vi "Read.vi"(8 "error in (no error)":errorcluster, 9 "Character Count":u32, 11 "VISA resource name in":refnum<visa-resource-name>) -> (0 "error out":errorcluster, 2 "Characters Read":string, 3 "VISA resource name out":refnum<visa-resource-name>)   [LabVIEW 2021, in "UART.lvlib"]
uses:
  <vilib>/myRIO/Instrument Drivers/Onboard IO/UART/UART.lvlib
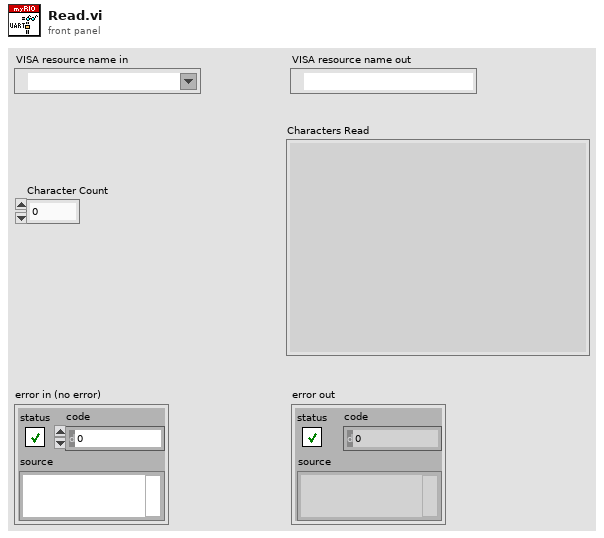
[diagram p1: front panel]
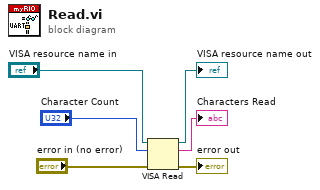
[diagram p0: block diagram]
diagram:
  n1 = VISA Read(VISA resource name="VISA resource name in", byte count="Character Count", error in (no error)="error in (no error)") -> (VISA resource name out=→"VISA resource name out":refnum<visa-resource-name>, read buffer=→"Characters Read":string, error out=→"error out":errorcluster)  [unwired: 1 out]
